vi "Hermite Interpolation 1D.vi"(9 "xi":dbl[](array[numeric]) format="%_6g", 10 "X":dbl[](array[numeric]), 11 "Y":dbl[](array[numeric])) -> (0 "error":i32, 1 "piecewise polynomial":T1 {"x locations" format="%.4g"; "coefficients" format="%.4g"}, 3 "yi":dbl[](array[numeric]) format="%_6g")   [LabVIEW 2018, in "NI_Gmath.lvlib"]
doc: "Performs one-dimensional interpolation using the cubic Hermite interpolation method based on the lookup table defined by <B>X</B> and <B>Y</B>."
uses:
  NI_Gmath.lvlib
  in_piecewise interp poly control.ctl
panel:
  # "Hermite Interpolation 1D"
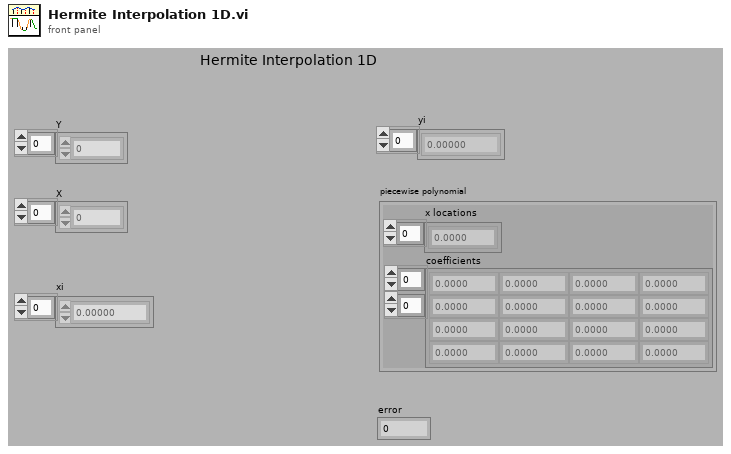
[diagram p1: front panel]
types:
  T1 = typedef "NI_Gmath.lvlib/in_piecewise interp poly control.ctl" = cluster{"x locations":dbl[], "coefficients":dbl[][]}
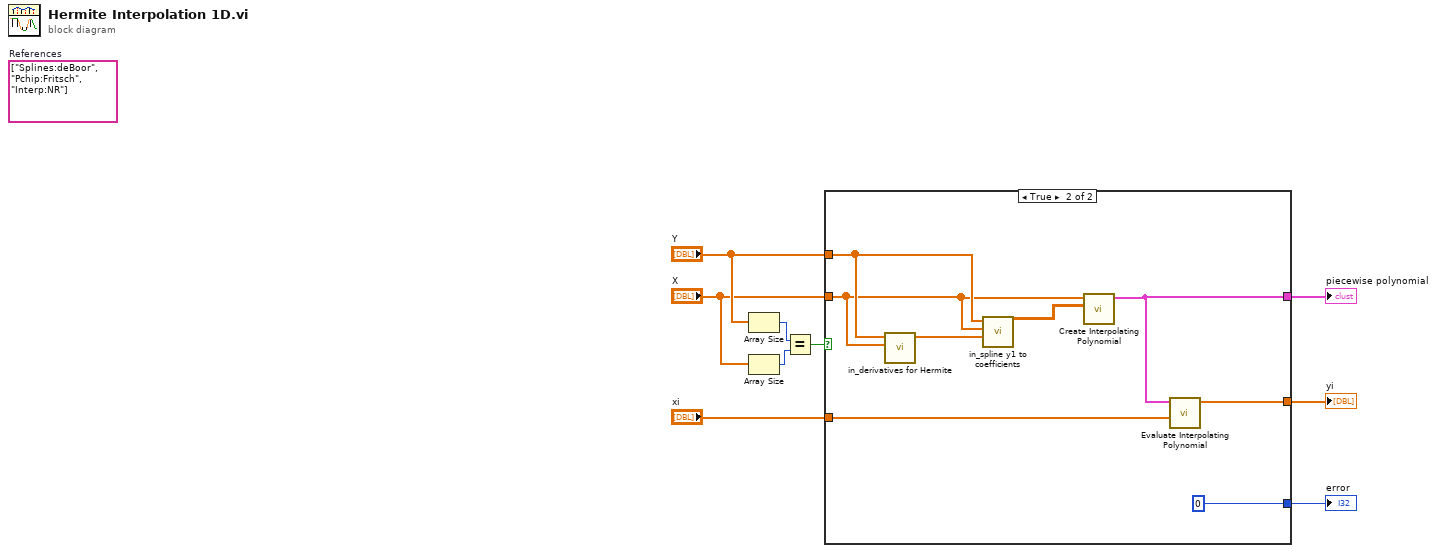
[diagram p0: block diagram]
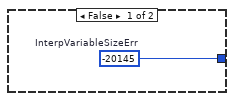
[diagram p2: hidden frame]
diagram:
  (unwired) string[] ["Splines:deBoor", "Pchip:Fritsch", "Interp:NR"]  # References
  n1 = Array Size(array="Y") -> (size(s)=w9:i32)
  n2 = Array Size(array="X") -> (size(s)=w8:i32)
  n3 = Equal?(x=w9, y=w8) -> (x = y?=w5:bool)
  n4 = case shown="True" w5 {
    tunnel: "Y" -> [_ w17]
    tunnel: "X" -> [_ w13]
    tunnel: [w10 0 ("error")] -> w4
    tunnel: "xi" -> [_ w15]
    tunnel: [_ w14] -> w2
    tunnel: [_ w11] -> w1
    frame False {
      w10 = -20145  # InterpVariableSizeErr
    }
    frame True {
      n5 = call "in_derivatives for Hermite.vi"("Y[0..N]"=w17, "X[0..N]"=w13) -> ("Y deriv[0..N]"=w18:dbl[])  [unwired: 8 in]
      n6 = call "in_spline y1 to coefficients.vi"("Y1"=w18, "X"=w13, "Y"=w17) -> ("coefficients"=w12:dbl[][])  [unwired: 8 in]
      n7 = call "Create Interpolating Polynomial.vi"("coefficients"=w12, "x locations"=w13) -> ("piecewise polynomial"=w11:T1)  [unwired: 8 in, 1 out]
      n8 = call "Evaluate Interpolating Polynomial.vi"("xi"=w15, "piecewise polynomial"=w11) -> ("yi"=w14:dbl[])  [unwired: 8 in, 1 out]
    }
  }
  "error" <- w4
  "yi" <- w2
  "piecewise polynomial" <- w1
